vi "Encode DM DATA.vi"(8 "error in (no error)":errorcluster, 10 "serial":string, 11 "Domino Laser module Class in":refnum<class "Domino Laser module Class.lvclass">) -> (0 "error out":errorcluster, 2 "DM":string, 3 "Domino Laser module Class out":refnum<class "Domino Laser module Class.lvclass">)   [LabVIEW 2015, in "Domino LM.lvlib" / "Domino Laser module Class.lvclass"]
uses:
  CTRLS/Domino Laser module Class.lvclass
  CTRLS/Open Batch Data.ctl
panel:
  in  "BatchData":T1
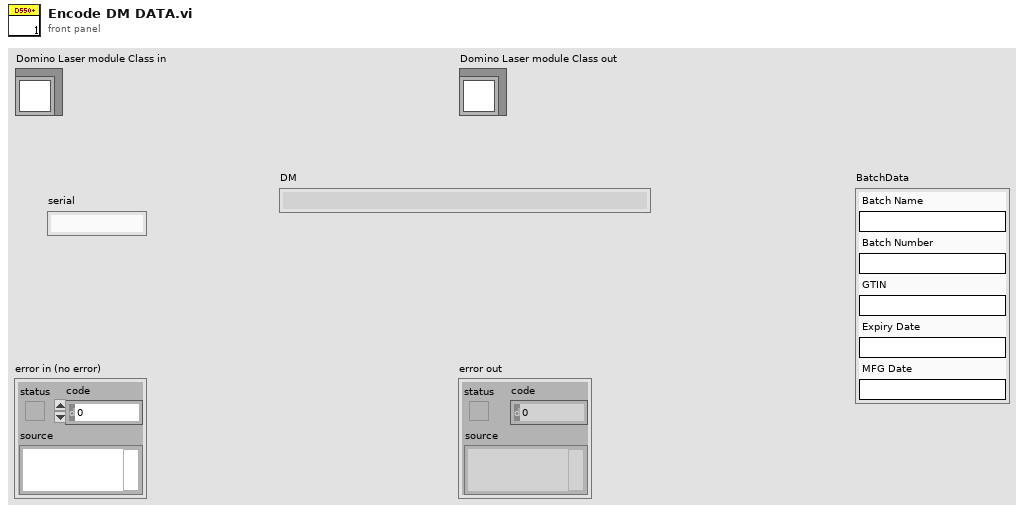
[diagram p1: front panel]
types:
  T1 = typedef "Open Batch Data.ctl" = cluster{"Batch Name":string, "Batch Number":string, "GTIN":string, "Expiry Date":string, "MFG Date":string}
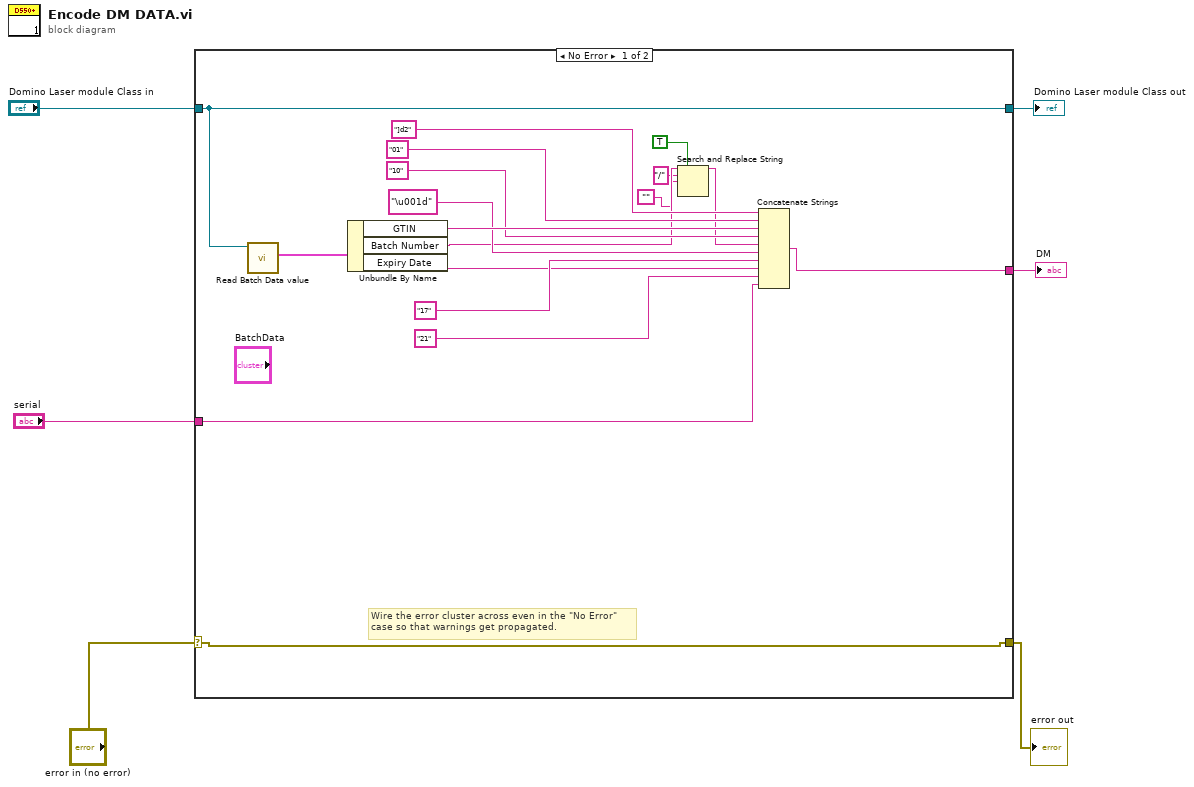
[diagram p0: block diagram]
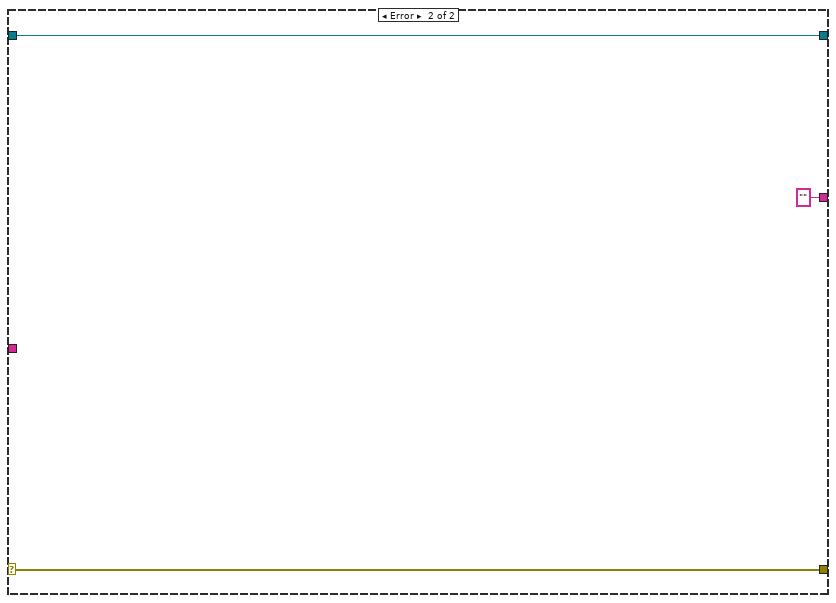
[diagram p2: hidden frame]
diagram:
  n1 = case shown="No Error" "error in (no error)" {
    selector: "error in (no error)" -> [w24 w27]
    tunnel: [w24 w27] -> w5
    tunnel: [w23 w26] -> w3
    tunnel: "Domino Laser module Class in" -> [w23 w26]
    tunnel: "serial" -> [w14 _]
    tunnel: [w13 ""] -> w1
    frame No Error {
      # "Wire the error cluster across even in the \"No Error\"\ncase so that warnings get propagated."
      n2 = call "Read Batch Data value.vi"("Domino Laser module Class in"=w23) -> ("Batch Data"=w22:T1)  [unwired: 8 in, 2 out]
      n3 = Unbundle By Name(w22) -> ("GTIN"=w20:string, "Batch Number"=w10:string, "Expiry Date"=w16:string)
      n4 = Search and Replace String(replace all?=TRUE ("replace all? (F)"), input string=w10, search string="/", replace string="") -> (result string=w9:string)  [unwired: 4 in, 3 out]
      n5 = Concatenate Strings("]d2" ("string"), "01" ("string"), w20, "10" ("string"), w9, "\u001d" ("string"), "17" ("string"), w16, "21" ("string"), w14) -> (w13:string)
    }
    frame Error {
    }
  }
  "error out" <- w5
  "Domino Laser module Class out" <- w3
  "DM" <- w1
